vi "Extract Basic Types Ctls.vi"(8 "error in (no error)":errorcluster, 11 "Ctls In":refnum<vi>[](array[refnum])) -> (0 "error out":errorcluster, 3 "Basic Types Ctls Out":refnum<vi>[](array[refnum]))   [LabVIEW 2020]
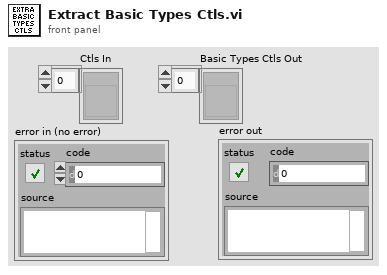
[diagram p1: front panel]
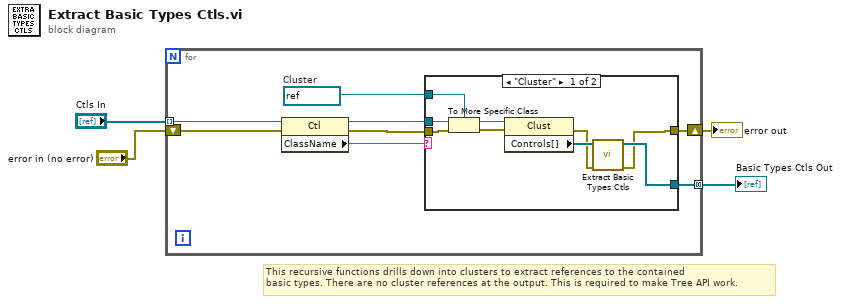
[diagram p0: block diagram]
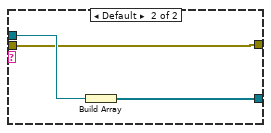
[diagram p2: hidden frame]
diagram:
  # "This recursive functions drills down into clusters to extract references to the contained\nbasic types. There are no cluster references at the output. This is required to make Tree API work."
  n1 = for {
    tunnel: "Ctls In" -> [w12] mode=indexing
    tunnel: [w9] -> w4 mode=concatenating
    shift-right: [w5] -> w1
    shift-left: "error in (no error)" -> [w7]
    w8 = refnum<vi> refnum  # Cluster
    n2 = property class="Ctl"(reference=w12, error in=w7) -> (reference out=w10:refnum<vi>, error out=w6:errorcluster, "ClassName"=w11:string)
    n3 = case shown="\"Cluster\"" w11 {
      tunnel: w10 -> [w21 w24]
      tunnel: [w17 w23] -> w9
      tunnel: w8 -> [w20 _]
      tunnel: w6 -> [w16 w22]
      tunnel: [w13 w22] -> w5
      frame "Cluster" {
        n4 = To More Specific Class(target class=w20, reference=w21, error in=w16) -> (specific class reference=w19:refnum<vi>, error out=w15:errorcluster)
        n5 = property class="Clust"(reference=w19, error in=w15) -> (error out=w14:errorcluster, "Controls[]"=w18:refnum<vi>[])  [unwired: 1 out]
        n6 = call <vilib>:"Extract Basic Types Ctls.vi"("error in (no error)"=w14, "Ctls In"=w18) -> ("error out"=w13:errorcluster, "Basic Types Ctls Out"=w17:refnum<vi>[])  [unwired: 8 in]
      }
      frame Default {
        n7 = Build Array(w24) -> (w23:refnum<vi>[])
      }
    }
  }
  "Basic Types Ctls Out" <- w4
  "error out" <- w1
